vi "set_params.vi"(0 "XPS in":refnum<class "XPS.lvclass">, 3 "error in (no error)":errorcluster) -> (7 "XPS out":refnum<class "XPS.lvclass">, 10 "error out":errorcluster)   [LabVIEW 2019, in "XPS.lvlib" / "XPS.lvclass"]
uses:
  XPS.lvclass
  XPS.lvclass/XPS.ctl
panel:
  in  "Group psoition name":string
  in  "Group name":string
  in  "stop":bool
  in  "pos_max":dbl[](array[numeric])
  # "Group1"
  # "Group1.Pos"
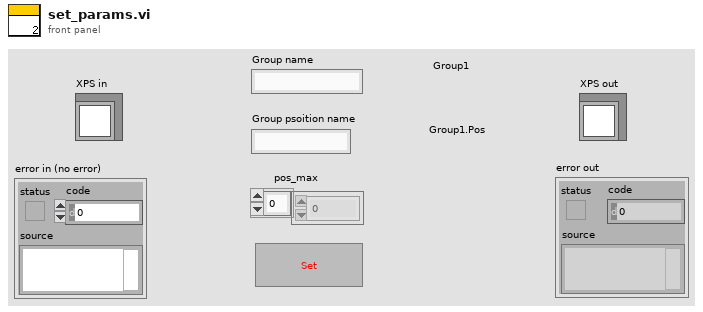
[diagram p1: front panel]
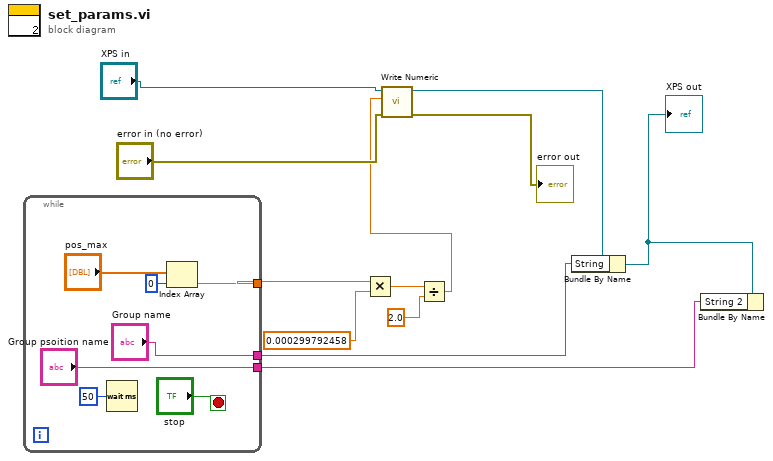
[diagram p0: block diagram]
diagram:
  n1 = while {
    tunnel: [w16] -> w9
    tunnel: ["Group name"] -> w3
    tunnel: ["Group psoition name"] -> w1
    stop <- "stop" stop-if-true
    n2 = Wait (ms)(milliseconds to wait=u32 50) -> ()  [unwired: 1 out]
    n3 = Index Array(array="pos_max", index=0) -> (element=w16:dbl)
  }
  n4 = Multiply(x=w9, y=0.000299792458) -> (x*y=w12:dbl)
  n5 = Divide(x=w12, y=2.0) -> (x/y=w5:dbl)
  n6 = call-dynamic "Write Numeric.vi"("error in (no error)"="error in (no error)", "Numeric"=w5, "XPS in"="XPS in") -> ("error out"=→"error out":errorcluster, "XPS out"=w4:refnum<class "XPS.lvclass">)  [unwired: 7 in]
  n7 = Bundle By Name(cluster=w4, "String"=w3) -> (w2:refnum<class "XPS.lvclass">)
  "XPS out" <- w2
  n8 = Bundle By Name(cluster=w2, "String 2"=w1) -> ()  [unwired: 1 out]
